vi "Read Setting_ver2.vi"(0 "configuration file path":path, 3 "error in (no error)":errorcluster) -> (6 "file path":path, 7 "output cluster 2":T1, 9 "error out":errorcluster)   [LabVIEW 2023]
uses:
  <vilib>/Utility/config.llb/Read Key (String).vi
  <vilib>/Utility/config.llb/Read Key (U32).vi
  <vilib>/Utility/config.llb/Read Key (Double).vi
  <vilib>/Utility/config.llb/Read Key (Path).vi
  <vilib>/Utility/config.llb/Read Key (I32).vi
  <vilib>/Utility/config.llb/NI_LVConfig.lvlib
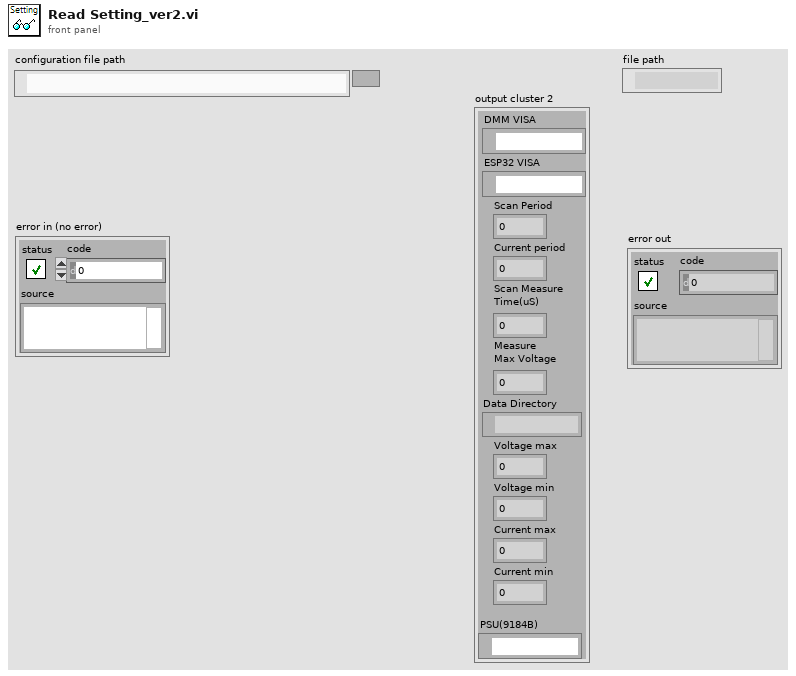
[diagram p1: front panel]
types:
  T1 = cluster{"DMM VISA":refnum<visa-resource-name>, "ESP32 VISA":refnum<visa-resource-name>, "Scan Period":u32, "Current period":u32, "Scan Measure\nTime(uS)":i32, "Measure\nMax Voltage":dbl, "Data Directory":path, "Voltage max":dbl, "Voltage min":dbl, "Current max":dbl, "Current min":dbl, "PSU(9184B)":refnum<visa-resource-name>}
  T2 = typedef "NI_LVConfig.lvlib/Config Data RefNum.ctl" = refnum<k1>
  T3 = cluster{"value":string, "value":string, "value":u32, "value":u32, "value":i32, "value":dbl, "value":path, "value":dbl, "value":dbl, "value":dbl, "value":dbl, "value":string}
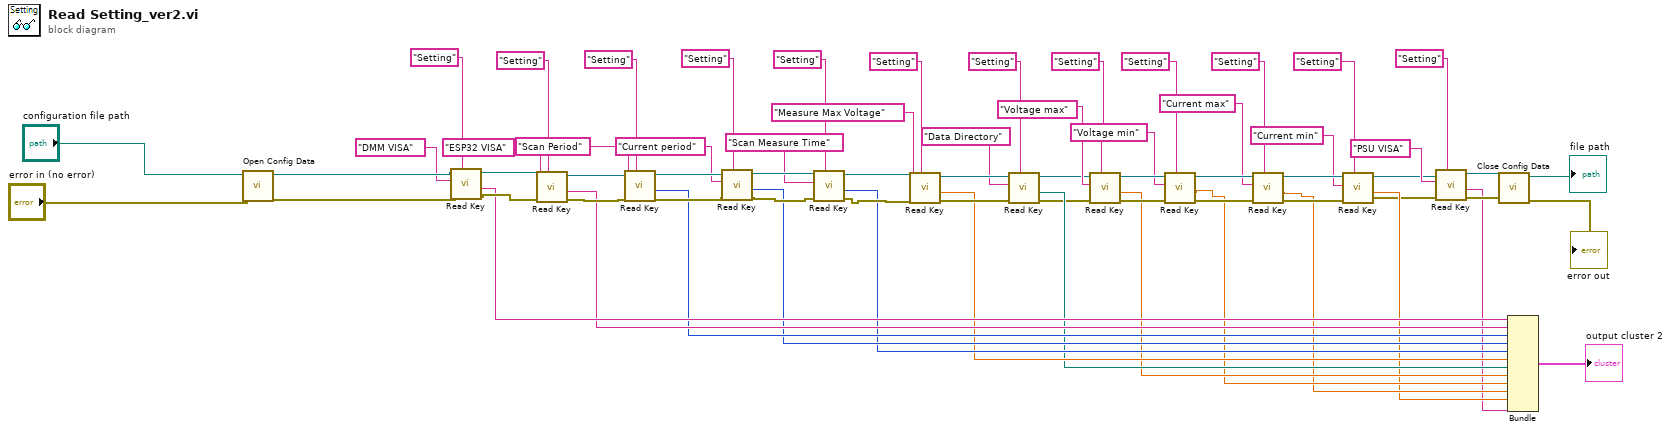
[diagram p0: block diagram]
diagram:
  n1 = call <vilib>:"Open Config Data.vi"("error in (no error)"="error in (no error)", "configuration file path"="configuration file path") -> ("error out"=w55:errorcluster, "refnum"=w56:T2)  [unwired: 7 in, 1 out]
  n2 = call-poly <vilib>:"Read Key.vi"("section"="Setting", "error in (no error)"=w55, "key"="DMM VISA", "refnum"=w56) -> ("error out"=w43:errorcluster, "value"=w35:string, "refnum out"=w54:T2)  [unwired: 4 in, 1 out]
  n3 = call-poly <vilib>:"Read Key.vi"("section"="Setting", "error in (no error)"=w43, "key"="ESP32 VISA", "refnum"=w54) -> ("error out"=w52:errorcluster, "value"=w34:string, "refnum out"=w53:T2)  [unwired: 4 in, 1 out]
  n4 = call-poly <vilib>:"Read Key.vi"("section"="Setting", "error in (no error)"=w52, "key"="Scan Period", "refnum"=w53) -> ("error out"=w50:errorcluster, "value"=w33:u32, "refnum out"=w51:T2)  [unwired: 4 in, 1 out]
  n5 = call-poly <vilib>:"Read Key.vi"("section"="Setting", "error in (no error)"=w50, "key"="Current period", "refnum"=w51) -> ("error out"=w48:errorcluster, "value"=w32:u32, "refnum out"=w49:T2)  [unwired: 4 in, 1 out]
  n6 = call-poly <vilib>:"Read Key.vi"("section"="Setting", "error in (no error)"=w48, "key"="Scan Measure Time", "refnum"=w49) -> ("error out"=w46:errorcluster, "value"=w31:i32, "refnum out"=w47:T2)  [unwired: 4 in, 1 out]
  n7 = call-poly <vilib>:"Read Key.vi"("section"="Setting", "error in (no error)"=w46, "key"="Measure Max Voltage", "refnum"=w47) -> ("error out"=w44:errorcluster, "value"=w30:dbl, "refnum out"=w45:T2)  [unwired: 4 in, 1 out]
  n8 = call-poly <vilib>:"Read Key.vi"("section"="Setting", "error in (no error)"=w44, "key"="Data Directory", "refnum"=w45) -> ("error out"=w13:errorcluster, "value"=w29:path, "refnum out"=w14:T2)  [unwired: 4 in, 1 out]
  n9 = call-poly <vilib>:"Read Key.vi"("section"="Setting", "error in (no error)"=w13, "key"="Voltage max", "refnum"=w14) -> ("error out"=w27:errorcluster, "value"=w12:dbl, "refnum out"=w28:T2)  [unwired: 4 in, 1 out]
  n10 = call-poly <vilib>:"Read Key.vi"("section"="Setting", "error in (no error)"=w27, "key"="Voltage min", "refnum"=w28) -> ("error out"=w25:errorcluster, "value"=w11:dbl, "refnum out"=w26:T2)  [unwired: 4 in, 1 out]
  n11 = call-poly <vilib>:"Read Key.vi"("section"="Setting", "error in (no error)"=w25, "key"="Current max", "refnum"=w26) -> ("error out"=w23:errorcluster, "value"=w10:dbl, "refnum out"=w24:T2)  [unwired: 4 in, 1 out]
  n12 = call-poly <vilib>:"Read Key.vi"("section"="Setting", "error in (no error)"=w23, "key"="Current min", "refnum"=w24) -> ("error out"=w4:errorcluster, "value"=w9:dbl, "refnum out"=w5:T2)  [unwired: 4 in, 1 out]
  n13 = call-poly <vilib>:"Read Key.vi"("section"="Setting", "error in (no error)"=w4, "key"="PSU VISA", "refnum"=w5) -> ("error out"=w2:errorcluster, "value"=w1:string, "refnum out"=w3:T2)  [unwired: 4 in, 1 out]
  n14 = call <vilib>:"Close Config Data.vi"("error in (no error)"=w2, "refnum"=w3) -> ("error out"=→"error out":errorcluster, "file path"=→"file path":path)  [unwired: 8 in]
  n15 = Bundle("value"=w35, "value"=w34, "value"=w33, "value"=w32, "value"=w31, "value"=w30, "value"=w29, "value"=w12, "value"=w11, "value"=w10, "value"=w9, "value"=w1) -> (→"output cluster 2":T3)  [unwired: 1 in]
